vi "Wait.vi"(8 "Error In":errorcluster, 11 "ms to wait":u32=20) -> (0 "Error Out":errorcluster)   [LabVIEW 2016]
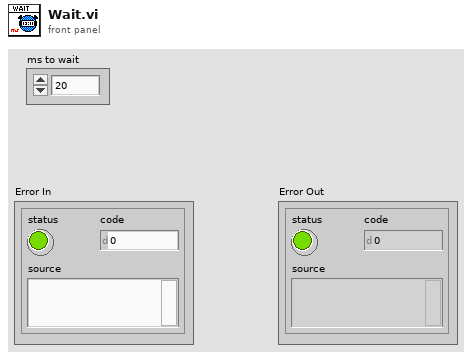
[diagram p1: front panel]
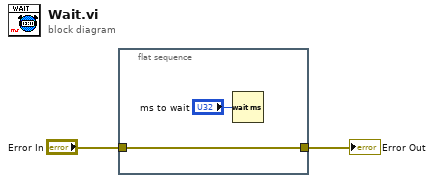
[diagram p0: block diagram]
diagram:
  n1 = flat-sequence {
    tunnel: [w3] -> w2
    tunnel: "Error In" -> [w3]
    frame #0 {
      n2 = Wait (ms)(milliseconds to wait="ms to wait") -> ()  [unwired: 1 out]
    }
  }
  "Error Out" <- w2
